vi "Get Joint Type.vi"(8 "error in (no error)":errorcluster, 11 "Link in":refnum<class "Link.lvclass">) -> (0 "error out":errorcluster, 2 "Joint Type":T1, 3 "Link out":refnum<class "Link.lvclass">)   [LabVIEW 2013, in "Link.lvclass"]
uses:
  Link.lvclass
  <vilib>/robotics/Kinematics/Link/Joint Type.ctl
  Link.lvclass/Link.ctl
  <vilib>/robotics/Kinematics/Link/NI_Robotics_Link.lvclass
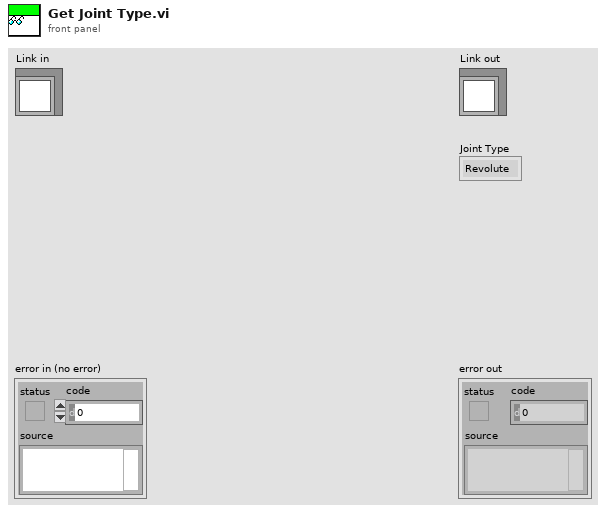
[diagram p1: front panel]
types:
  T1 = typedef "NI_Robotics_Link.lvclass/Joint Type.ctl" = enum16{"Revolute", "Prismatic"}
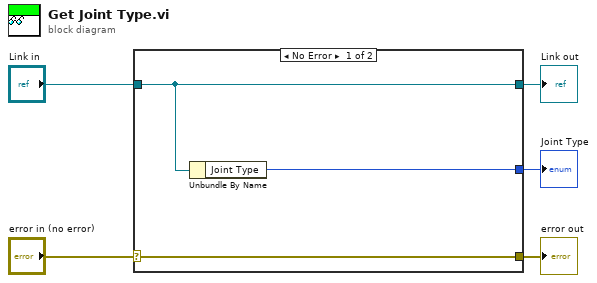
[diagram p0: block diagram]
diagram:
  n1 = case shown="No Error" "error in (no error)" {
    selector: "error in (no error)" -> [w8 w9]
    tunnel: [w8 w9] -> w4
    tunnel: [w7 w10] -> w2
    tunnel: "Link in" -> [w7 w10]
    tunnel: [w6 _] -> w1
    frame No Error {
      n2 = Unbundle By Name(w7) -> ("Joint Type"=w6:T1)
    }
    frame Error {
    }
  }
  "error out" <- w4
  "Link out" <- w2
  "Joint Type" <- w1
